vi "PH_BeamlineInformation.get Head Index by in Use Service Name.vi"(0 "i ref in":refnum<vi>, 2 "In Use Service Name":string, 5 "error in (no error)":errorcluster) -> (13 "current in use linked?":bool, 14 "i ref out":refnum<vi>, 16 "index of element":i32, 17 "in Use GUI Ref":refnum<vi>, 18 "current in use value":bool, 19 "error out":errorcluster)   [LabVIEW 2014, in "PH_BeamlineInformation.lvlib"]
uses:
  PH_BeamlineInformation.lvlib
  PH_Basics/PH_PowerUnit_BaseClass/PH_PowerUnit_BaseClass.PP PU Tags.ctl
  PH_Basics/PH_PowerUnit_BaseClass/PH_PowerUnit_BaseClass.lvlib
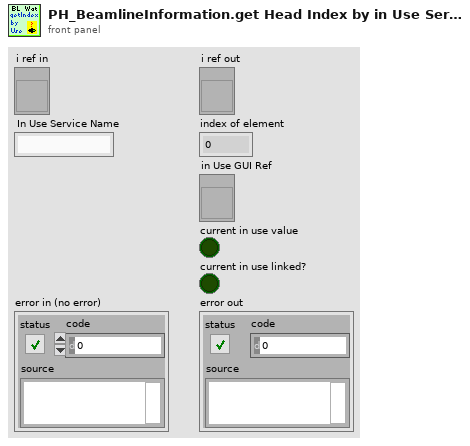
[diagram p1: front panel]
types:
  T1 = typedef "PH_PowerUnit_BaseClass.lvlib/PH_PowerUnit_BaseClass.PP PU Tags.ctl" = enum16{"Waiting-Time", "PU-in-Use"}
  T2 = typedef "PH_BeamlineInformation.lvlib/PH_BeamlineInformation.i attribute.ctl" = cluster{"BL GUI Elements of Services":cluster{"Service Name":string, "GUI Elements":refnum<vi>[], "Status":i32}[], "Powermeters":T3, "Efficiency":T4, "Heads":T5[]}
  T3 = typedef "PH_BeamlineInformation.lvlib/PH_BeamlineInformation.Powermeter.ctl" = cluster{"ns FE":cluster{"GUI Ref":refnum<vi>, "Value":dbl}, "fs FE":cluster{"GUI Ref":refnum<vi>, "Value":dbl}, "PA":cluster{"GUI Ref":refnum<vi>, "Value":dbl}, "MA":cluster{"GUI Ref":refnum<vi>, "Value":dbl}, "Z6 green":cluster{"GUI Ref":refnum<vi>, "Value":dbl}, "Z6 IR":cluster{"GUI Ref":refnum<vi>, "Value":dbl}, "Z6 COS":cluster{"GUI Ref":refnum<vi>, "Value":dbl}}
  T4 = typedef "PH_BeamlineInformation.lvlib/PH_BeamlineInformation.Efficiency.ctl" = cluster{"PA Gain":cluster{"GUI Ref":refnum<vi>, "Value":dbl}, "MA Gain":cluster{"GUI Ref":refnum<vi>, "Value":dbl}, "Z6 green Conversion":cluster{"GUI Ref":refnum<vi>, "Value":dbl}, "Z6 Comp Losses":cluster{"GUI Ref":refnum<vi>, "Value":dbl}}
  T5 = typedef "PH_BeamlineInformation.lvlib/PH_BeamlineInformation.Head.ctl" = cluster{"PowerUnit":T6, "in use":cluster{"Value":bool, "GUI Ref":refnum<vi>, "linked":bool}, "voltage":cluster{"Value":dbl, "GUI Ref":refnum<vi>, "linked":bool}}
  T6 = typedef "PH_PP_Common.lvlib/PH_PP_Common.PUs.ctl" = enum16{"no Info", "PA-19mm-1", "PA-19mm-2", "PA-45mm-PILC", "PA-45mm-MAIN", "MA-PU-1", "MA-PU-2", "MA-PU-3", "MA-PU-4", "MA-PU-5", "MA-PU-6", "MA-FR", "MA-PILC", "PA-45mm-DP"}
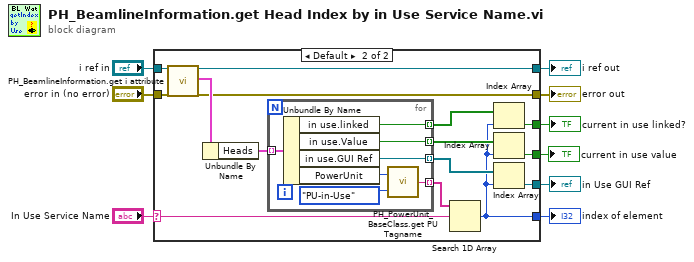
[diagram p0: block diagram]
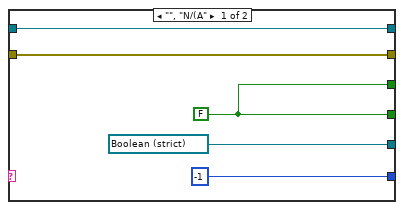
[diagram p2: hidden frame]
diagram:
  n1 = case shown="Default" "In Use Service Name" {
    selector: "In Use Service Name" -> [_ w24]
    tunnel: [w14 w27] -> w9
    tunnel: "i ref in" -> [w14 w26]
    tunnel: [-1 ("index of element") w16] -> w7
    tunnel: "error in (no error)" -> [w13 w25]
    tunnel: [w13 w19] -> w5
    tunnel: [refnum<vi> refnum ("GUI Ref") w22] -> w3
    tunnel: [w10 w20] -> w2
    tunnel: [w10 w15] -> w1
    frame "", "N/(A" {
      w10 = FALSE ("in use")
    }
    frame Default {
      n2 = call "PH_BeamlineInformation.get i attribute.vi"("i ref in"=w26, "error in (no error)"=w25) -> ("i ref out"=w27:refnum<vi>, "i attribute"=w28:T2, "error out"=w19:errorcluster)  [unwired: 15 in]
      n3 = Unbundle By Name(w28) -> ("Heads"=w18:T5[])
      n4 = for {
        tunnel: w18 -> [w36] mode=indexing
        tunnel: [w32] -> w29 mode=indexing
        tunnel: [w35] -> w23 mode=indexing
        tunnel: [w34] -> w21 mode=indexing
        tunnel: [w30] -> w17 mode=indexing
        n5 = Unbundle By Name(w36) -> ("in use.linked"=w30:bool, "in use.Value"=w34:bool, "in use.GUI Ref"=w35:refnum<vi>, "PowerUnit"=w33:T6)
        n6 = call "PH_PowerUnit_BaseClass.get PU Tagname.vi"("PU Tag"=PH_PowerUnit_BaseClass.PP_PU_Tags."PU-in-Use", "PU"=w33) -> ("PU Tagname"=w32:string)
      }
      n7 = Search 1D Array(1D array=w29, element=w24) -> (index of element=w16:i32)  [unwired: 1 in]
      n8 = Index Array(array=w17, index=w16) -> (element=w15:bool)
      n9 = Index Array(array=w21, index=w16) -> (element=w20:bool)
      n10 = Index Array(array=w23, index=w16) -> (element=w22:refnum<vi>)
    }
  }
  "i ref out" <- w9
  "error out" <- w5
  "index of element" <- w7
  "in Use GUI Ref" <- w3
  "current in use value" <- w2
  "current in use linked?" <- w1
